vi "DRAM FIFO Pattern Checker.vi"(8 "Input Valid":bool, 11 "Input Data":T1) -> (0 "Points Done":u32, 1 "Pattern Match Ever Fail?":bool, 2 "Last Address Failed":u32, 3 "Pattern Match Failed?":bool, 4 "Expected Data":u64, 5 "Bank0.Failed FIFO Data":u64, 7 "Bank1. Failed FIFO Data":u64)   [LabVIEW 2011]
uses:
  Data Type (256).ctl
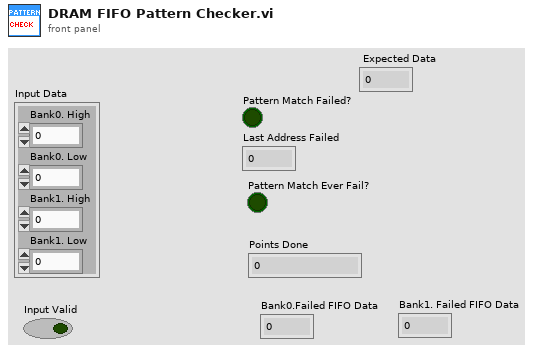
[diagram p1: front panel]
types:
  T1 = typedef "Data Type (256).ctl" = cluster{"Bank0. High":u64, "Bank0. Low":u64, "Bank1. High":u64, "Bank1. Low":u64}
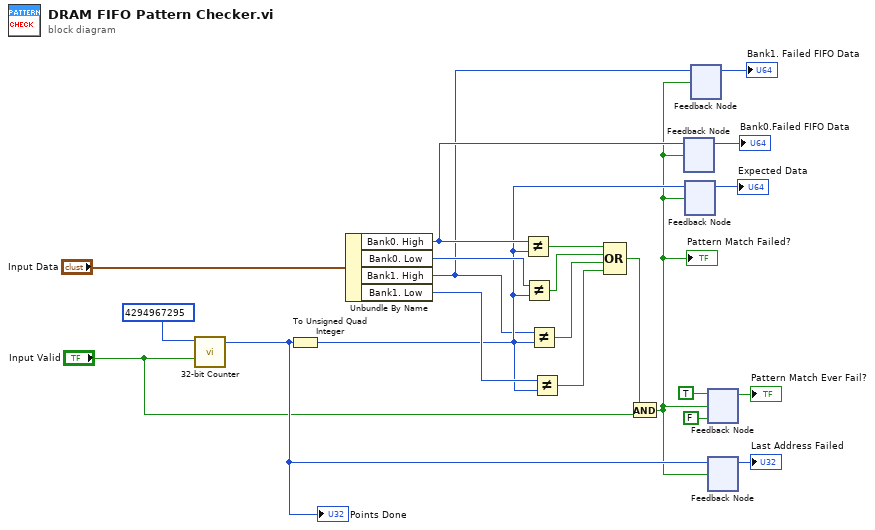
[diagram p0: block diagram]
diagram:
  n1 = call "32-bit Counter.vi"("INC?"="Input Valid", "rollover"=u32 4294967295) -> ("count"=w14:u32)  [unwired: 9 in]
  "Points Done" <- w14
  n2 = To Unsigned Quad Integer(1:w14) -> (0:w5:u64)
  n3 = Unbundle By Name("Input Data") -> ("Bank0. High"=w7:u64, "Bank0. Low"=w20:u64, "Bank1. High"=w2:u64, "Bank1. Low"=w19:u64)
  n4 = Not Equal?(x=w7, y=w5) -> (x != y?=w18:bool)
  n5 = Not Equal?(x=w20, y=w5) -> (x != y?=w17:bool)
  n6 = Not Equal?(x=w2, y=w5) -> (x != y?=w16:bool)
  n7 = Not Equal?(x=w19, y=w5) -> (x != y?=w15:bool)
  n8 = Compound Arithmetic op=OR(w18, w17, w16, w15) -> (w9:bool)
  n9 = And(x=w9, y="Input Valid") -> (x .and. y?=w1:bool)
  "Pattern Match Failed?" <- w1
  n10 = feedback #1() -> (→"Bank0.Failed FIFO Data":u64)  [unwired: 1 in]
  n11 = feedback-in #1(w7, w1) -> ()
  n12 = feedback #2() -> (→"Expected Data":u64)  [unwired: 1 in]
  n13 = feedback-in #2(w5, w1) -> ()
  n14 = feedback #3() -> (→"Bank1. Failed FIFO Data":u64)  [unwired: 1 in]
  n15 = feedback-in #3(w2, w1) -> ()
  n16 = feedback #4(FALSE) -> (→"Pattern Match Ever Fail?":bool)
  n17 = feedback-in #4(TRUE, w1) -> ()
  n18 = feedback-in #5(w14, w1) -> ()
  n19 = feedback #5() -> (→"Last Address Failed":u32)  [unwired: 1 in]
